vi "Config_General.vi"() -> ()   [LabVIEW 2015]
panel:
  out "output array":string[](array[string])
  in  "RX_DIGFIL_PD":bool
  out "com_temp":string[](array[string])
  out "实时信息":string="*IDN?"
  in  "stop 9":bool
  in  "stop 8":bool
  in  "stop 7":bool
  in  "stop 6":bool
  in  "stop 5":bool
  in  "stop 4":bool
  in  "stop 3":bool
  in  "stop 2":bool
  in  "stop":bool
  in  "TXVGA":bool
  in  "RXLOBUF":bool
  in  "LNA":bool
  in  "MIX":bool
  in  "TA":bool
  in  "RX_FRONT":bool
  in  "CKPATH":bool
  in  "TX":bool
  in  "RX":bool
  in  "TXPLL":bool
  in  "RXPLL":bool
  in  "BBPLL":bool
  in  "外部10M信号":dbl
  in  "OK Button":bool
  in  "测试报告路径":path
  in  "配置文件路径":path
  in  "测试人员ID":string="001"
  out "?":string="#"
  out "?":string="测试人员ID"
  in  "芯片ID":string="123456789"
  out "?":string="#"
  out "?":string="芯片ID"
  out "?":string="#"
  in  "测试板ID":dbl=4.0
  out "?":string="测试板ID"
  out "?":string="℃"
  in  "环境温度":dbl=24.0
  out "?":string="环境温度"
  in  "b1 13":bool
  in  "RXVGA":bool
  in  "PA":bool
  in  "DAC":bool
  in  "ADC":bool
  in  "DAC CLK DIV":enum16{"DIV/0", "DIV/2", "DIV/4"}(ring)
  in  "ADC CLK DIV":enum16{"DIV/0", "DIV/2", "DIV/4"}(ring)
  in  "RXPLL DIV":enum16{"DIV/0", "DIV/2", "DIV/4"}(ring)
  in  "TXPLL DIV":enum16{"DIV/0", "DIV/2", "DIV/4"}(ring)
  in  "VSA":enum16{""}(ring)
  in  "b1 11":bool
  in  "VSA":enum16{""}(ring)
  in  "DAC_EXT_CLK(M)":dbl
  in  "DAC_EXT_CLK(M)":bool
  in  "DAC BBPLL":bool
  in  "ADC_EXT_CLK":dbl
  in  "ADC BBPLL":bool
  in  "ADC_EXT_CLK(M)":bool
  in  "b1 6":bool
  in  "TX_EXT_LO(M)":dbl
  in  "TXPLL":bool
  in  "TX_EXT_LO(M)":bool
  in  "RX_EXT_LO(M)":dbl
  in  "RXPLL":bool
  in  "RX_EXT_LO(M)":bool
  in  "VSA":enum16{""}(ring)
  in  "b1 2":bool
  in  "信号源":enum16{""}(ring)
  # "MIXER"
  # "VGA"
  # "ADC"
  # "LNA"
  # "A/D CLK SEL"
  # "RX CLK SEL"
  # "RXPLL"
  # "BBPLL"
  # "TX CLK SEL"
  # "D/A CLK SEL"
  # "TXPLL"
  # "PA"
  # "VGA"
  # "DAC"
  # "MIXER"
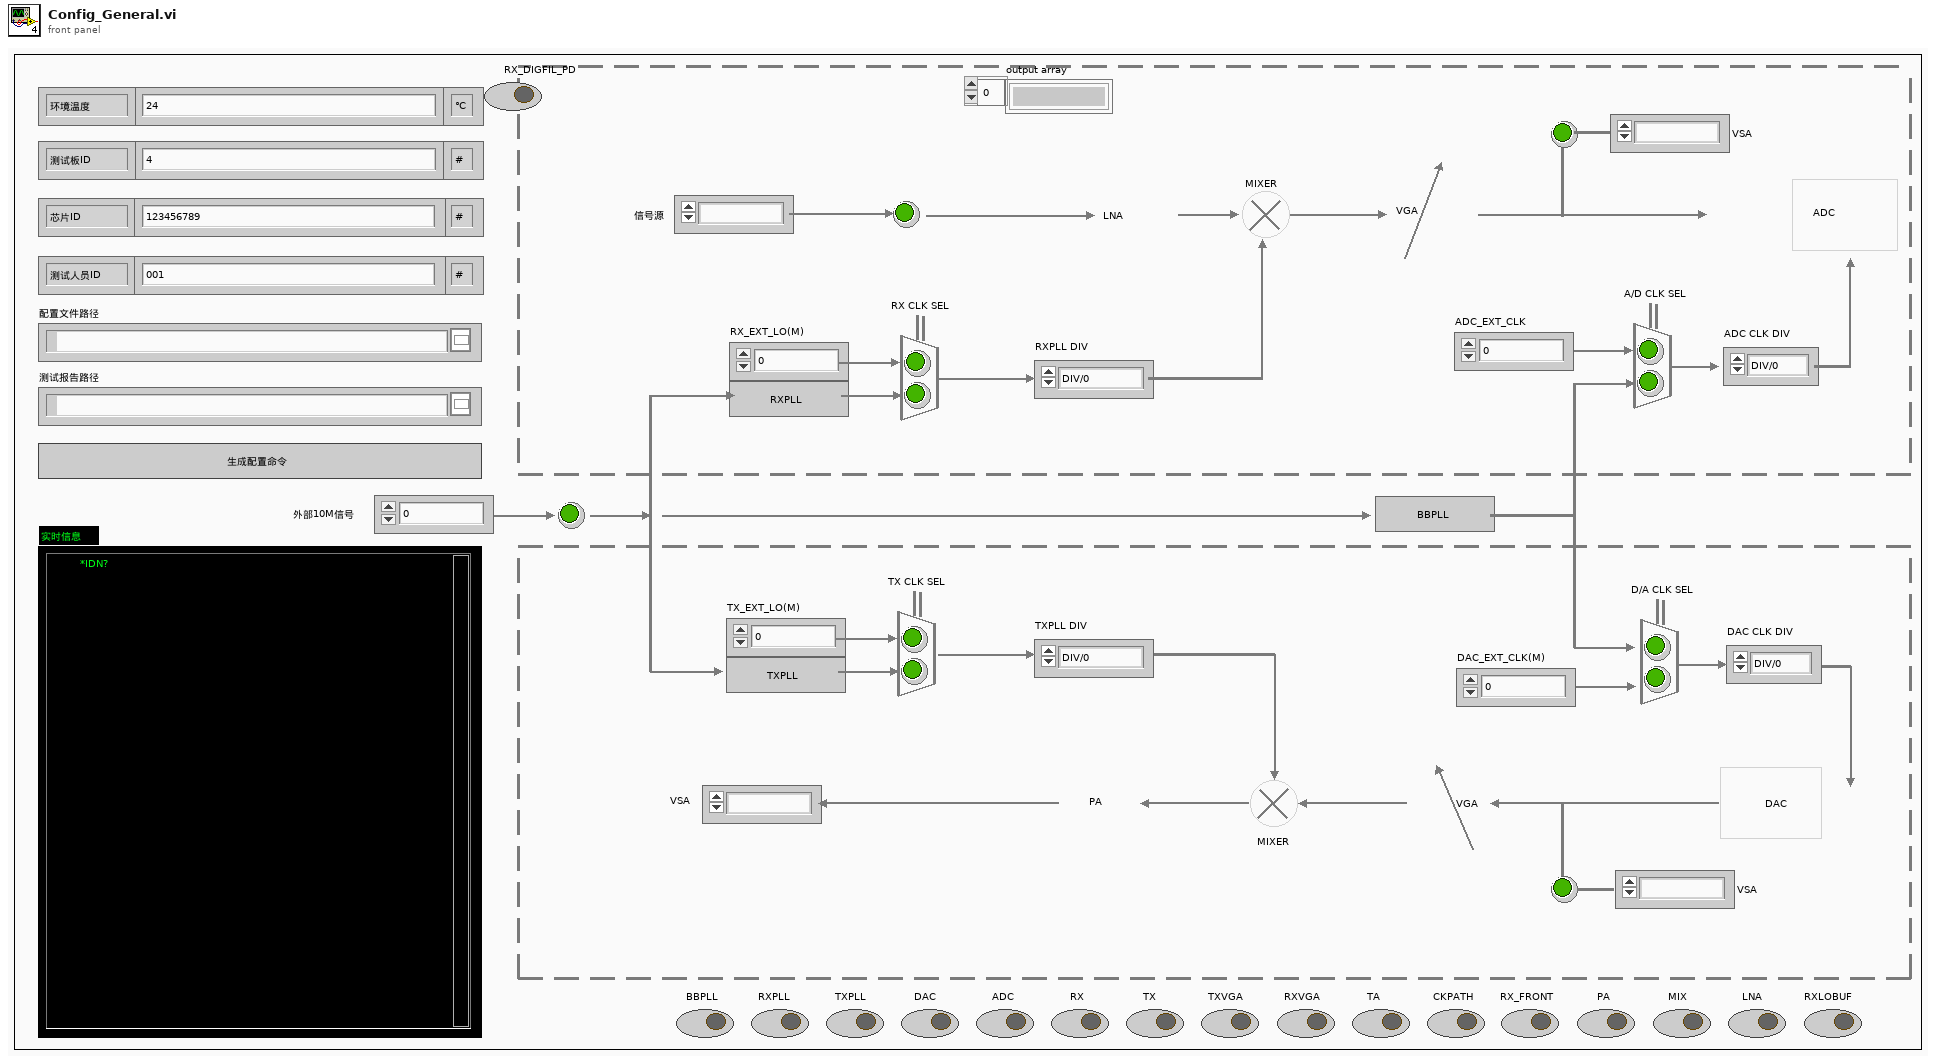
[diagram p1: front panel]
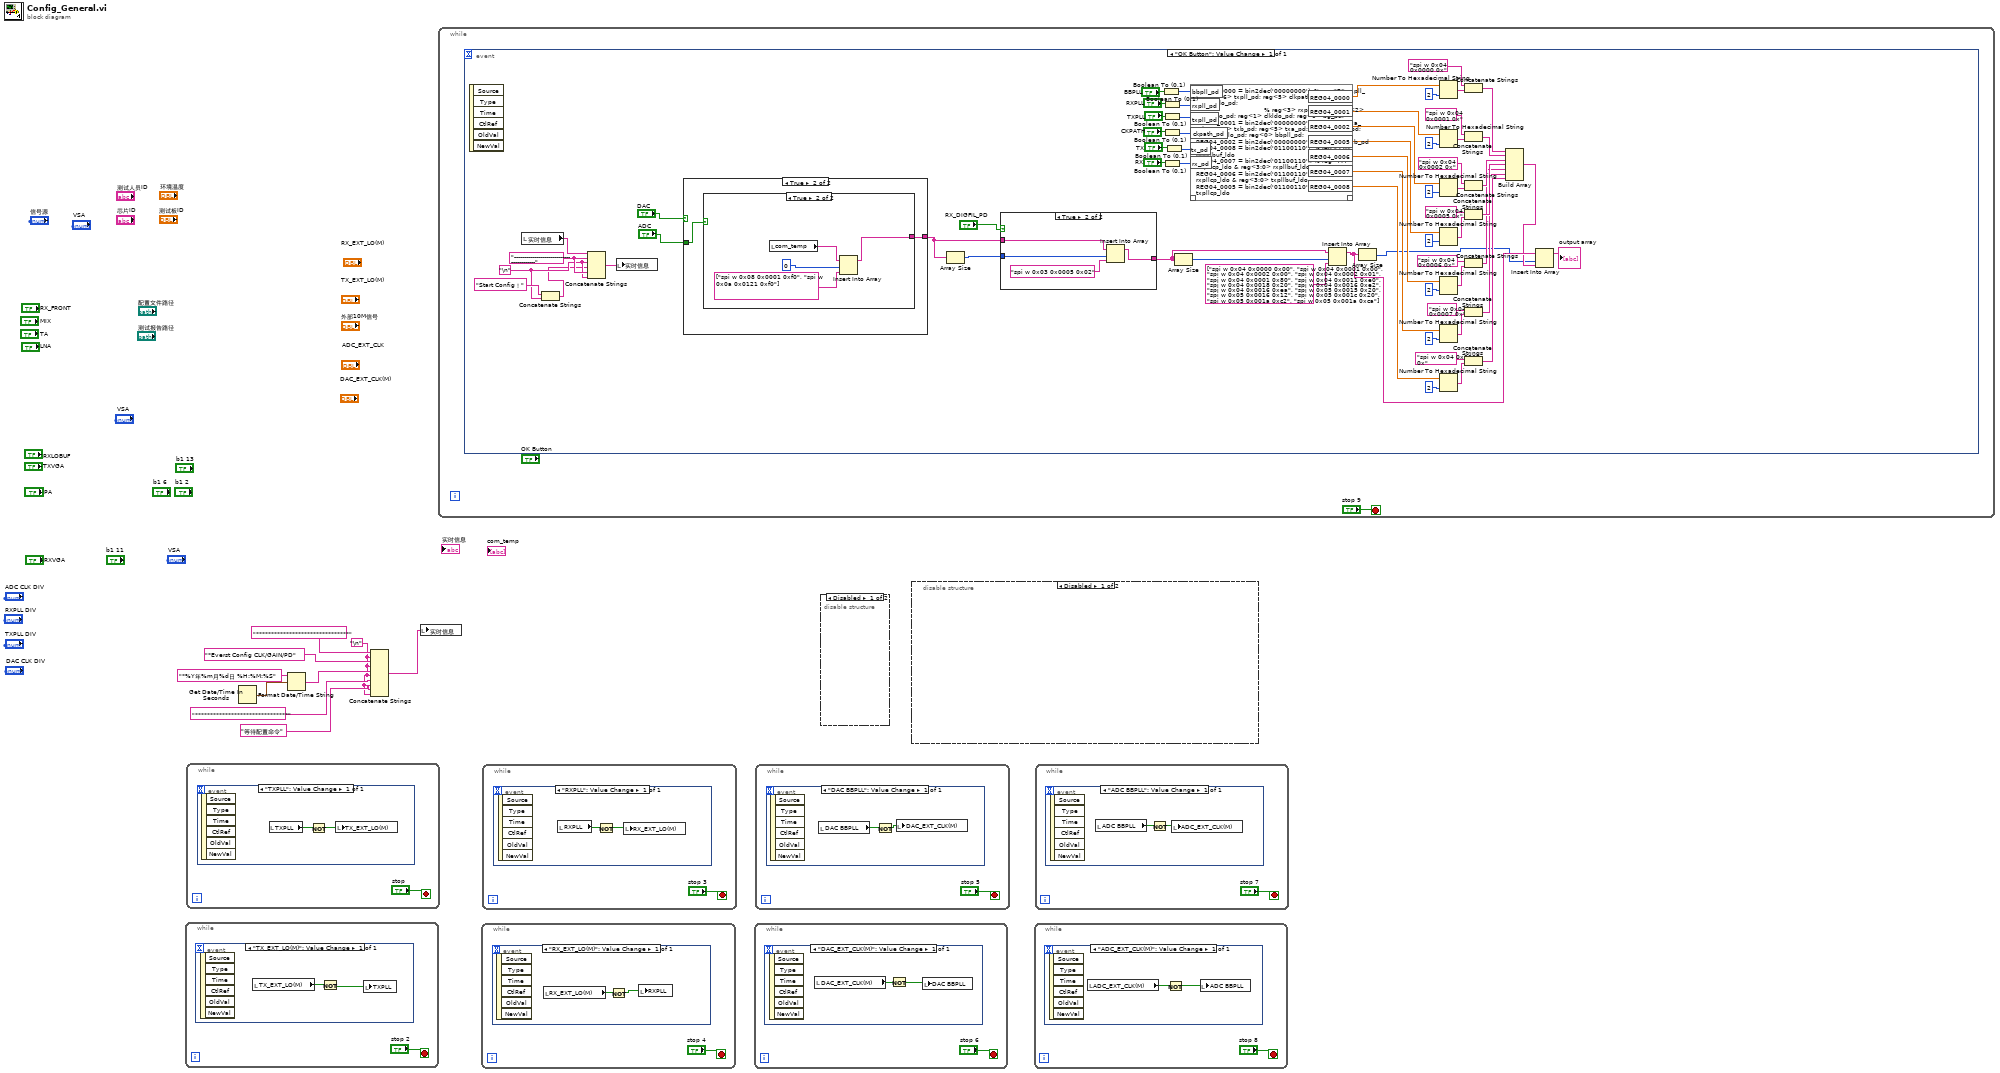
[diagram p0: block diagram]
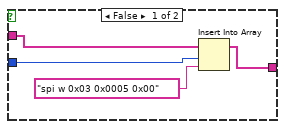
[diagram p2: hidden frame]
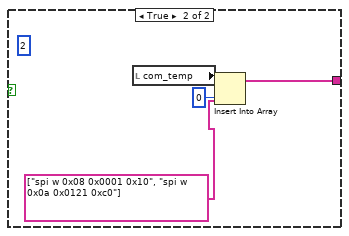
[diagram p4: hidden frame]
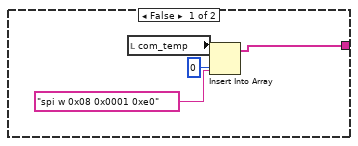
[diagram p5: hidden frame]
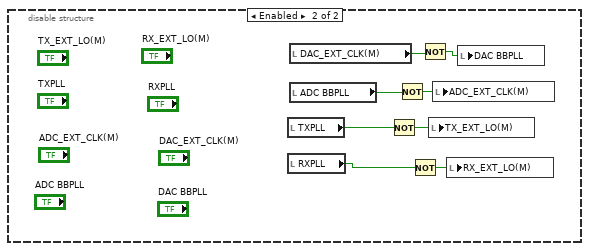
[diagram p6: hidden frame]
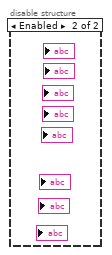
[diagram p7: hidden frame]
diagram:
  w1 = "\n"
  n1 = while {
    stop <- "stop 2" stop-if-true
    n2 = event shown="[0] \"TX_EXT_LO(M)\": Value Change" {
      selector: _ -> [_]
      dyn-events: _ -> [_]
      timeout: _ -> [_]
      event "TX_EXT_LO(M)": Value Change {
        n3 = event-data() -> ()  [unwired: 1 in, 6 out]
        n4 = local read "TX_EXT_LO(M)"() -> (w11:bool)
        n5 = Not(x=w11) -> (.not. x?=w12:bool)
        n6 = local write "TXPLL"(w12) -> ()
      }
    }
  }
  n7 = while {
    stop <- "stop" stop-if-true
    n8 = event shown="[0] \"TXPLL\": Value Change" {
      selector: _ -> [_]
      dyn-events: _ -> [_]
      timeout: _ -> [_]
      event "TXPLL": Value Change {
        n9 = event-data() -> ()  [unwired: 1 in, 6 out]
        n10 = local read "TXPLL"() -> (w15:bool)
        n11 = Not(x=w15) -> (.not. x?=w14:bool)
        n12 = local write "TX_EXT_LO(M)"(w14) -> ()
      }
    }
  }
  n13 = Get Date/Time In Seconds() -> (seconds since 1Jan1904=w6:timestamp)
  n14 = Format Date/Time String(time format string (%c)="*%Y年%m月%d日 %H:%M:%S", seconds (now)=w6) -> (date/time string=w5:string)  [unwired: 1 in]
  n15 = Concatenate Strings("*******************************" ("string"), w1, "*Everst Config CLK/GAIN/PD" ("string"), w1, w5, w1, "*******************************" ("string"), w1, "等待配置命令" ("string"), w1) -> (w4:string)
  n16 = local write "实时信息"(w4) -> ()
  n17 = while {
    stop <- "stop 9" stop-if-true
    n18 = event shown="[0] \"OK Button\": Value Change" {
      selector: _ -> [_]
      dyn-events: _ -> [_]
      timeout: _ -> [_]
      event "OK Button": Value Change {
        w78 = "\n"
        w80 = "----------------------------------------" ("string")
        n19 = event-data() -> ()  [unwired: 1 in, 6 out]
        n20 = local read "实时信息"() -> (w81:string)
        n21 = Concatenate Strings("Start Config！" ("string"), w78) -> (w77:string)
        n22 = Concatenate Strings(w81, w80, w78, w77, w80, w78) -> (w74:string)
        n23 = local write "实时信息"(w74) -> ()
        n24 = case shown="True" "DAC" {
          tunnel: "ADC" -> [w91 w97]
          tunnel: [w90 w96] -> w71
          frame False {
            n25 = case shown="False" w91 {
              tunnel: [_ w92] -> w90
              frame False {
              }
              frame True {
                (unwired) 2
                n26 = local read "com_temp"() -> (w94:string[])
                n27 = Insert Into Array(array=w94, index=0, new element=string[] ["spi w 0x08 0x0001 0x10", "spi w 0x0a 0x0121 0xc0"]) -> (w92:string[])
              }
            }
          }
          frame True {
            n28 = case shown="True" w97 {
              tunnel: [w98 w103] -> w96
              frame False {
                n29 = local read "com_temp"() -> (w101:string[])
                n30 = Insert Into Array(array=w101, index=0, new element="spi w 0x08 0x0001 0xe0" ("往芯片写数据")) -> (w98:string[])
              }
              frame True {
                n31 = local read "com_temp"() -> (w105:string[])
                n32 = Insert Into Array(array=w105, index=0, new element=string[] ["spi w 0x08 0x0001 0xf0", "spi w 0x0a 0x0121 0xf0"]) -> (w103:string[])
              }
            }
          }
        }
        n33 = Array Size(array=w71) -> (size(s)=w72:i32)
        n34 = case shown="True" "RX_DIGFIL_PD" {
          tunnel: w72 -> [w84 w89]
          tunnel: w71 -> [w83 w87]
          tunnel: [w82 w86] -> w56
          frame False {
            n35 = Insert Into Array(array=w83, index=w84, new element="spi w 0x03 0x0005 0x00" ("往芯片写数据")) -> (w82:string[])
          }
          frame True {
            n36 = Insert Into Array(array=w87, index=w89, new element="spi w 0x03 0x0005 0x02" ("往芯片写数据")) -> (w86:string[])
          }
        }
        n37 = Boolean To (0,1)(Boolean="BBPLL") -> (0, 1=w59:i16)
        n38 = Boolean To (0,1)(Boolean="RXPLL") -> (0, 1=w60:i16)
        n39 = Boolean To (0,1)(Boolean="TXPLL") -> (0, 1=w61:i16)
        n40 = Boolean To (0,1)(Boolean="CKPATH") -> (0, 1=w62:i16)
        n41 = Boolean To (0,1)(Boolean="RX") -> (0, 1=w64:i16)
        n42 = Boolean To (0,1)(Boolean="TX") -> (0, 1=w63:i16)
        n43 = Array Size(array=w56) -> (size(s)=w57:i32)
        n44 = script code="REG04_0000 = bin2dec('00000000'); % reg<7> rxpll_pd; reg<6> txpll_pd; reg<5> clkpath_pd; reg<4> bbpll_ldo_pd;\n                                  % reg<3> rxpll_ldo_pd; reg<2> txpll_ldo_pd; reg<1> clkldo_pd; reg<0> bg_pd;\nREG04_0001 = bin2dec('00000000'); % reg<7> rxa_pd; reg<6> txb_pd; reg<5> txa_pd; reg<2> rxlo_pd; reg<1> txlo_pd; reg<0> bbpll_pd;\nREG04_0002 = bin2dec('00000000'); % reg<0> rxb_pd\nREG04_0008 = bin2dec('01100110'); % reg<3:0> bbpllbuf_ldo\nREG04_0007 = bin2dec('01100110'); % reg<7:4> bbpllcp_ldo & reg<3:0> rxpllbuf_ldo\nREG04_0006 = bin2dec('01100110'); % reg<7:4> rxpllcp_ldo & reg<3:0> txpllbuf_ldo\nREG04_0005 = bin2dec('01100110'); % reg<7:4> txpllcp_ldo\n\n\nif bbpll_pd\n    REG04_0000 = bitor(bin2dec('00010000'),REG04_0000);\n    REG04_0001 = bitor(bin2dec('00000001'),REG04_0001);\n    REG04_0007 = bitor(bin2dec('00010000'),REG04_0007);\n    REG04_0008 = bitor(bin2dec('00000001'),REG04_0008);\nend\n\nif rxpll_pd\n    REG04_0000 = bitor(bin2dec('10001000'),REG04_0000);\n    REG04_0006 = bitor(bin2dec('00010000'),REG04_0006);\nend\n\nif txpll_pd\n    REG04_0000 = bitor(bin2dec('01000100'),REG04_0000);\n    REG04_0005 = bitor(bin2dec('00010000'),REG04_0005);\n    REG04_0006 = bitor(bin2dec('00000001'),REG04_0006);\nend\n\nif ckpath_pd\n    REG04_0000 = bitor(bin2dec('00100000'),REG04_0000);\n    REG04_0005 = bitor(bin2dec('00000001'),REG04_0005);\nend\n\nif tx_pd\n    REG04_0001 = bitor(bin2dec('01100000'),REG04_0001);\nend\n\nif rx_pd\n    REG04_0001 = bitor(bin2dec('10000000'),REG04_0001);\n    REG04_0002 = bitor(bin2dec('00000001'),REG04_0002);\nend"("bbpll_pd"=w59, "rxpll_pd"=w60, "txpll_pd"=w61, "ckpath_pd"=w62, "tx_pd"=w63, "rx_pd"=w64) -> ("REG04_0000"=w27:dbl, "REG04_0001"=w26:dbl, "REG04_0002"=w25:dbl, "REG04_0005"=w24:dbl, "REG04_0006"=w23:dbl, "REG04_0007"=w22:dbl, "REG04_0008"=w21:dbl)  [unwired: 1 in, 1 out]
        n45 = Insert Into Array(array=w56, index=w57, new element=string[] ["spi w 0x04 0x0000 0x00", "spi w 0x04 0x0001 0x00", "spi w 0x04 0x0002 0x00", "spi w 0x04 0x0002 0x01", "spi w 0x04 0x0001 0x80", "spi w 0x04 0x0011 0xe0", "spi w 0x04 0x0018 0x20", "spi w 0x04 0x0016 0xe2", "spi w 0x04 0x0016 0xea", "spi w 0x05 0x0015 0x20", "spi w 0x05 0x0016 0x12", "spi w 0x05 0x001c 0x20", "spi w 0x05 0x001a 0xc2", "spi w 0x05 0x001a 0xca"]) -> (w20:string[])
        n46 = Array Size(array=w20) -> (size(s)=w18:i32)
        n47 = Number To Hexadecimal String(1:i16 2 ("宽度(-)"), 2:w27) -> (0:w47:string)
        n48 = Number To Hexadecimal String(1:i16 2 ("宽度(-)"), 2:w26) -> (0:w39:string)
        n49 = Number To Hexadecimal String(1:i16 2 ("宽度(-)"), 2:w25) -> (0:w46:string)
        n50 = Number To Hexadecimal String(1:i16 2 ("宽度(-)"), 2:w24) -> (0:w38:string)
        n51 = Number To Hexadecimal String(1:i16 2 ("宽度(-)"), 2:w23) -> (0:w44:string)
        n52 = Number To Hexadecimal String(1:i16 2 ("宽度(-)"), 2:w22) -> (0:w35:string)
        n53 = Number To Hexadecimal String(1:i16 2 ("宽度(-)"), 2:w21) -> (0:w41:string)
        n54 = Concatenate Strings("spi w 0x04 0x0000 0x", w47) -> (w34:string)
        n55 = Concatenate Strings("spi w 0x04 0x0001 0x", w39) -> (w33:string)
        n56 = Concatenate Strings("spi w 0x04 0x0002 0x", w46) -> (w32:string)
        n57 = Concatenate Strings("spi w 0x04 0x0005 0x", w38) -> (w31:string)
        n58 = Concatenate Strings("spi w 0x04 0x0006 0x", w44) -> (w30:string)
        n59 = Concatenate Strings("spi w 0x04 0x0007 0x", w35) -> (w29:string)
        n60 = Concatenate Strings("spi w 0x04 0x0008 0x", w41) -> (w28:string)
        n61 = Build Array(w34, w33, w32, w31, w30, w29, w28) -> (w19:string[])
        n62 = Insert Into Array(array=w20, index=w18, new element=w19) -> (→"output array":string[])
      }
    }
  }
  n63 = while {
    stop <- "stop 4" stop-if-true
    n64 = event shown="[0] \"RX_EXT_LO(M)\": Value Change" {
      selector: _ -> [_]
      dyn-events: _ -> [_]
      timeout: _ -> [_]
      event "RX_EXT_LO(M)": Value Change {
        n65 = event-data() -> ()  [unwired: 1 in, 6 out]
        n66 = local read "RX_EXT_LO(M)"() -> (w107:bool)
        n67 = Not(x=w107) -> (.not. x?=w108:bool)
        n68 = local write "RXPLL"(w108) -> ()
      }
    }
  }
  n69 = while {
    stop <- "stop 3" stop-if-true
    n70 = event shown="[0] \"RXPLL\": Value Change" {
      selector: _ -> [_]
      dyn-events: _ -> [_]
      timeout: _ -> [_]
      event "RXPLL": Value Change {
        n71 = event-data() -> ()  [unwired: 1 in, 6 out]
        n72 = local read "RXPLL"() -> (w111:bool)
        n73 = Not(x=w111) -> (.not. x?=w110:bool)
        n74 = local write "RX_EXT_LO(M)"(w110) -> ()
      }
    }
  }
  n75 = while {
    stop <- "stop 6" stop-if-true
    n76 = event shown="[0] \"DAC_EXT_CLK(M)\": Value Change" {
      selector: _ -> [_]
      dyn-events: _ -> [_]
      timeout: _ -> [_]
      event "DAC_EXT_CLK(M)": Value Change {
        n77 = event-data() -> ()  [unwired: 1 in, 6 out]
        n78 = local read "DAC_EXT_CLK(M)"() -> (w113:bool)
        n79 = Not(x=w113) -> (.not. x?=w114:bool)
        n80 = local write "DAC BBPLL"(w114) -> ()
      }
    }
  }
  n81 = while {
    stop <- "stop 5" stop-if-true
    n82 = event shown="[0] \"DAC BBPLL\": Value Change" {
      selector: _ -> [_]
      dyn-events: _ -> [_]
      timeout: _ -> [_]
      event "DAC BBPLL": Value Change {
        n83 = event-data() -> ()  [unwired: 1 in, 6 out]
        n84 = local read "DAC BBPLL"() -> (w116:bool)
        n85 = Not(x=w116) -> (.not. x?=w117:bool)
        n86 = local write "DAC_EXT_CLK(M)"(w117) -> ()
      }
    }
  }
  n87 = disable-structure shown="Disabled" {
    frame Disabled {
    }
    frame Enabled {
    }
  }
  n88 = disable-structure shown="Disabled" {
    frame Disabled {
    }
    frame Enabled {
      n89 = local read "TXPLL"() -> (w122:bool)
      n90 = local read "RXPLL"() -> (w121:bool)
      n91 = local read "DAC_EXT_CLK(M)"() -> (w124:bool)
      n92 = local read "ADC BBPLL"() -> (w123:bool)
      n93 = Not(x=w122) -> (.not. x?=w119:bool)
      n94 = Not(x=w123) -> (.not. x?=w125:bool)
      n95 = Not(x=w121) -> (.not. x?=w120:bool)
      n96 = Not(x=w124) -> (.not. x?=w118:bool)
      n97 = local write "TX_EXT_LO(M)"(w119) -> ()
      n98 = local write "ADC_EXT_CLK(M)"(w125) -> ()
      n99 = local write "RX_EXT_LO(M)"(w120) -> ()
      n100 = local write "DAC BBPLL"(w118) -> ()
    }
  }
  n101 = while {
    stop <- "stop 8" stop-if-true
    n102 = event shown="[0] \"ADC_EXT_CLK(M)\": Value Change" {
      selector: _ -> [_]
      dyn-events: _ -> [_]
      timeout: _ -> [_]
      event "ADC_EXT_CLK(M)": Value Change {
        n103 = event-data() -> ()  [unwired: 1 in, 6 out]
        n104 = local read "ADC_EXT_CLK(M)"() -> (w128:bool)
        n105 = Not(x=w128) -> (.not. x?=w127:bool)
        n106 = local write "ADC BBPLL"(w127) -> ()
      }
    }
  }
  n107 = while {
    stop <- "stop 7" stop-if-true
    n108 = event shown="[0] \"ADC BBPLL\": Value Change" {
      selector: _ -> [_]
      dyn-events: _ -> [_]
      timeout: _ -> [_]
      event "ADC BBPLL": Value Change {
        n109 = event-data() -> ()  [unwired: 1 in, 6 out]
        n110 = local read "ADC BBPLL"() -> (w130:bool)
        n111 = Not(x=w130) -> (.not. x?=w131:bool)
        n112 = local write "ADC_EXT_CLK(M)"(w131) -> ()
      }
    }
  }
